vi "Get Type.vi"(11 "Double 1D in":refnum<class "Double 1D.lvclass">) -> (3 "Type":string)   [LabVIEW 2020, in "Double 1D.lvclass"]
uses:
  <vilib>/gpm_packages/@cs/data-type-serializer/source/Double 1D/Double 1D.lvclass
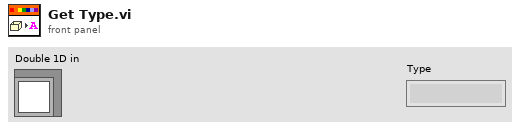
[diagram p1: front panel]
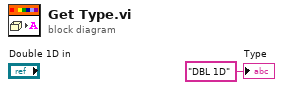
[diagram p0: block diagram]
diagram:
  "Type" <- "DBL 1D" ("Type")
